vi "SysDef.Item.Remove.vi"(8 "error in (no error)":errorcluster, 11 "nodeID":u64) -> (0 "error out":errorcluster, 1 "Removed":bool)   [LabVIEW 2016, in "Advanced System Definition.lvlib"]
uses:
  Advanced System Definition.lvlib
  NationalInstruments.VeriStand.SystemDefinitionAPI
  <vilib>/NI VeriStand/Custom Device API/Custom Device API.lvlib
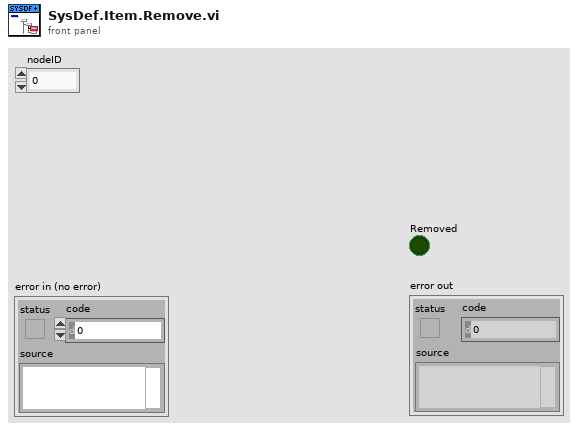
[diagram p1: front panel]
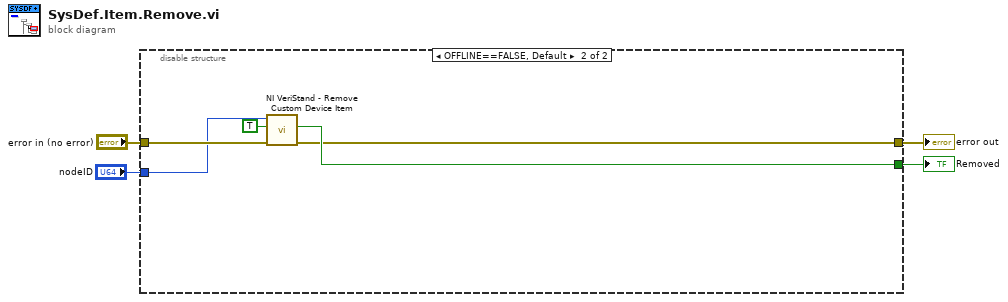
[diagram p0: block diagram]
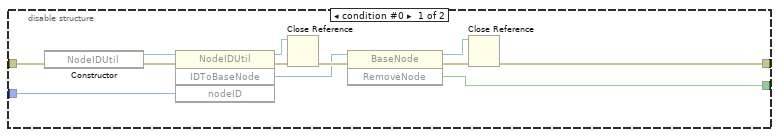
[diagram p2: hidden frame]
diagram:
  n1 = disable-structure shown="OFFLINE==FALSE, Default" {
    disable-tunnel: [w6 w18] -> w4
    disable-tunnel: [w8 w19] -> w3
    disable-tunnel: "error in (no error)" -> [w14 w21]
    disable-tunnel: "nodeID" -> [w11 w20]
    frame condition #0 {
      n2 = constructor class="NodeIDUtil"(error in=w14) -> (reference out=w16:refnum<k24>, error out=w15:errorcluster)  [unwired: 2 in, 1 out]
      n3 = invoke class="NodeIDUtil" method="IDToBaseNode"(reference=w16, error in=w15, "nodeID"=w11) -> (reference out=w13:refnum<k24>, error out=w12:errorcluster, "IDToBaseNode"=w9:refnum<k24>)  [unwired: 1 in, 1 out]
      n4 = Close Reference(reference=w13, error in (no error)=w12) -> (error out=w10:errorcluster)
      n5 = invoke class="BaseNode" method="RemoveNode"(reference=w9, error in=w10) -> (reference out=w5:refnum<k24>, error out=w7:errorcluster, "RemoveNode"=w8:bool)  [unwired: 1 in]
      n6 = Close Reference(reference=w5, error in (no error)=w7) -> (error out=w6:errorcluster)
    }
    frame condition #1 (active) {
      n7 = call <vilib>:"NI VeriStand - Remove Custom Device Item.vi"("error in (no error)"=w21, "Force Delete (F)"=TRUE, "Item Ref in"=w20) -> ("error out"=w18:errorcluster, "Deleted?"=w19:bool)  [unwired: 7 in]
    }
  }
  "error out" <- w4
  "Removed" <- w3
